vi "Auto Processing Level.vi"(7 "Reset? (F)":bool, 8 "Debounce Period (5s)":dbl=5.0, 9 "Period (0.1s)":dbl=0.1 format="%#_13g", 11 "#Left In Q":i32) -> (0 "Since Upgraded (s)":dbl, 2 "LogInQ Changing Speed (#/s)":dbl, 3 "Level":T1)   [LabVIEW 2017, in "Communicable State Machine.lvlib"]
doc: "Dynamically calculates the recommended log processing level based on the current number of logs in the global log queue.\n\n-- <b>Controls</b> --\n- <b>#Left In Q</b>: Number of remaining logs in the global log queue.\n- <b>Debounce Period (5s)</b>: Log processing upgrade time. If logs in the global log queue consistently increase within the specified time, the processing level will be upgraded.\n- <b>Period (0.1s)</b>: Detection period. The default is 100 ms.\n- <b>Reset? (F)</b>: Reset flag.\n\n-- <b>Indicators</b> --\n- <b>Level</b>: Processing level. \"Normal\" indicates standard processing. Higher levels omit different information to increase processing speed.\n- <b>LogInQ Changing Speed (#/s)</b>: Current rate of log change in the global log queue.\n- <b>Since Upgraded (S)</b>: Time since the last processing level upgrade."
uses:
  Communicable State Machine.lvlib
  _support/Periodic String Filter Level.ctl
  _Shared/CSM Shared.lvlib
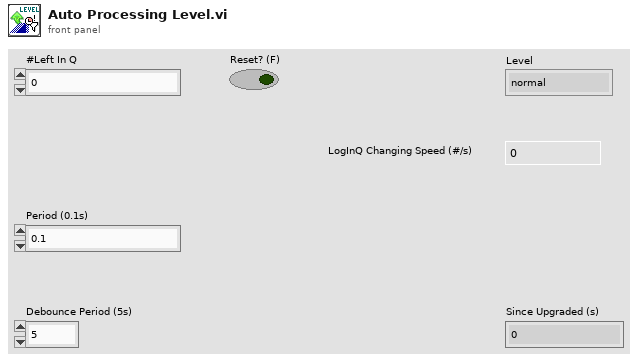
[diagram p1: front panel]
types:
  T1 = typedef "Communicable State Machine.lvlib/Periodic String Filter Level.ctl" = enum16{"normal", "L1", "L2", "L3", "L4"}
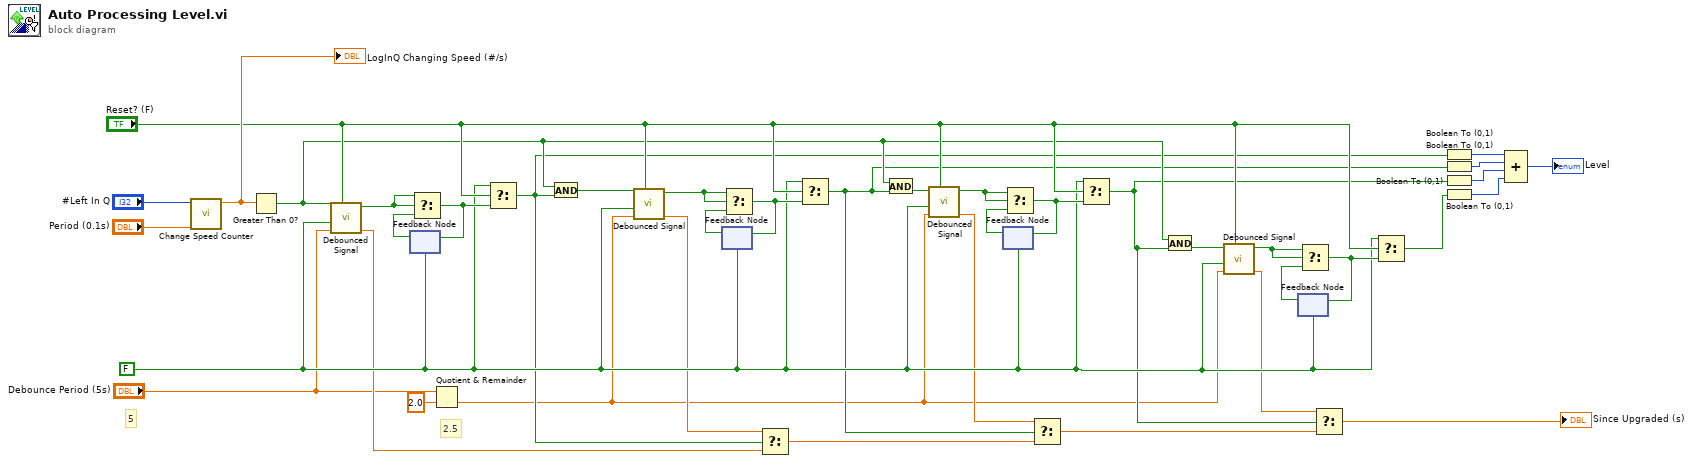
[diagram p0: block diagram]
diagram:
  w20 = FALSE ("reset value")
  # "2.5"
  # "5"
  n1 = call "Change Speed Counter.vi"("Period (0.1s)"="Period (0.1s)", "Numeric"="#Left In Q") -> ("Speed (#/s)"=w38:dbl)  [unwired: 7 in, 2 out]
  "LogInQ Changing Speed (#/s)" <- w38
  n2 = Greater Than 0?(x=w38) -> (x > 0?=w15:bool)
  n3 = call "Debounced Signal.vi"("Reset? (F)"="Reset? (F)", "Debounce Period (5s)"="Debounce Period (5s)", "Reset Value"=w20, "Signal"=w15) -> ("Since Last Change (S)"=w8:dbl, "Signal (Safe)"=w39:bool)  [unwired: 6 in]
  n4 = feedback #1(w20) -> (w40:bool)
  n5 = Select(t=w39, s=w39, f=w40) -> (s? t:f=w35:bool)
  n6 = feedback-in #1(w35) -> ()
  n7 = Quotient & Remainder(x="Debounce Period (5s)", y=2.0) -> (floor(x/y)=w1:dbl)  [unwired: 1 out]
  n8 = Select(t=w20, s="Reset? (F)", f=w35) -> (s? t:f=w10:bool)
  n9 = And(x=w15, y=w10) -> (x .and. y?=w18:bool)
  n10 = call "Debounced Signal.vi"("Reset? (F)"="Reset? (F)", "Debounce Period (5s)"=w1, "Reset Value"=w20, "Signal"=w18) -> ("Since Last Change (S)"=w6:dbl, "Signal (Safe)"=w32:bool)  [unwired: 6 in]
  n11 = feedback #2(w20) -> (w33:bool)
  n12 = Select(t=w32, s=w32, f=w33) -> (s? t:f=w34:bool)
  n13 = feedback-in #2(w34) -> ()
  n14 = Select(t=w6, s=w10, f=w8) -> (s? t:f=w9:dbl)
  n15 = Select(t=w20, s="Reset? (F)", f=w34) -> (s? t:f=w14:bool)
  n16 = And(x=w15, y=w14) -> (x .and. y?=w17:bool)
  n17 = call "Debounced Signal.vi"("Reset? (F)"="Reset? (F)", "Debounce Period (5s)"=w1, "Reset Value"=w20, "Signal"=w17) -> ("Since Last Change (S)"=w5:dbl, "Signal (Safe)"=w29:bool)  [unwired: 6 in]
  n18 = feedback #3(w20) -> (w31:bool)
  n19 = Select(t=w29, s=w29, f=w31) -> (s? t:f=w30:bool)
  n20 = feedback-in #3(w30) -> ()
  n21 = Select(t=w5, s=w14, f=w9) -> (s? t:f=w12:dbl)
  n22 = Select(t=w20, s="Reset? (F)", f=w30) -> (s? t:f=w13:bool)
  n23 = And(x=w15, y=w13) -> (x .and. y?=w16:bool)
  n24 = call "Debounced Signal.vi"("Reset? (F)"="Reset? (F)", "Debounce Period (5s)"=w1, "Reset Value"=w20, "Signal"=w16) -> ("Since Last Change (S)"=w4:dbl, "Signal (Safe)"=w24:bool)  [unwired: 6 in]
  n25 = feedback #4(w20) -> (w22:bool)
  n26 = Select(t=w24, s=w24, f=w22) -> (s? t:f=w23:bool)
  n27 = feedback-in #4(w23) -> ()
  n28 = Select(t=w4, s=w13, f=w12) -> (s? t:f=→"Since Upgraded (s)":dbl)
  n29 = Select(t=w20, s="Reset? (F)", f=w23) -> (s? t:f=w11:bool)
  n30 = Boolean To (0,1)(Boolean=w10) -> (0, 1=w28:i16)
  n31 = Boolean To (0,1)(Boolean=w14) -> (0, 1=w27:i16)
  n32 = Boolean To (0,1)(Boolean=w13) -> (0, 1=w26:i16)
  n33 = Boolean To (0,1)(Boolean=w11) -> (0, 1=w19:i16)
  n34 = Compound Arithmetic op=ADD(w28, w27, w26, w19) -> (→"Level":i16)
